vi "Search_From_Json.vi"(0 "Data JSON":string, 7 "ERD":string, 11 "error in":errorcluster) -> (4 "Name":string, 6 "Type":string, 8 "Size data":string, 10 "Hexa":string, 15 "error IO":errorcluster)   [LabVIEW 2021]
uses:
  <vilib>/JDP Science/JSONtext/Find Item.vi
  <vilib>/JDP Science/JSONtext/String Subset.vi
  <vilib>/JDP Science/JSONtext/Offset/Find Object Item Locations by Names.vi
  <vilib>/JDP Science/JSONtext/support/Quote and Escape JSON string.vi
  <vilib>/JDP Science/JSONtext/Next JSON Value.vi
  <vilib>/JDP Science/JSONtext/Parsing/Advance past whitespace.vi
  <vilib>/JDP Science/JSONtext/support/Commas Needed.vi
  <vilib>/JDP Science/JSONtext/Parsing/Advance past whitespace and comma.vi
  <vilib>/JDP Science/JSONtext/Parsing/Advance past next JSON Value (inlined COPY).vi
  <vilib>/JDP Science/JSONtext/Parsing/Advance past Item Name.vi
  <vilib>/JDP Science/JSONtext/support/quote and escape json string 2.vi
  <vilib>/JDP Science/JSONtext/Parsing/Advance past Line Ending.vi
  <vilib>/JDP Science/JSONtext/Parsing/Advance past String.vi
  <vilib>/JDP Science/JSONtext/Parsing/Advance past Number.vi
  <vilib>/JDP Science/JSONtext/Parsing/Parse Full Path or Item Name.vi
  <vilib>/JDP Science/JSONtext/Parsing/Advance past Array.vi
  <vilib>/JDP Science/JSONtext/Parsing/Advance past Object.vi
  <vilib>/JDP Science/JSONtext/support/Error Cluster From Code.vi
  <vilib>/JDP Science/JSONtext/Offset/Find Item Locations by Path.vi
  <vilib>/JDP Science/JSONtext/Parsing/Parsing Error.vi
  <vilib>/JDP Science/JSONtext/JSONtext.lvlib
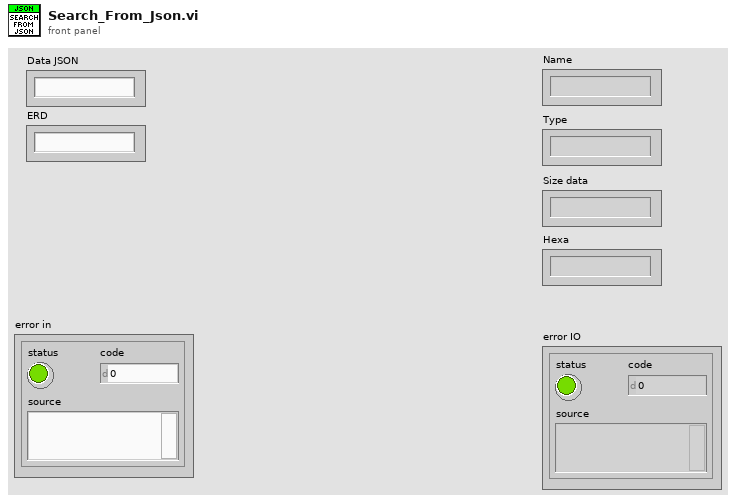
[diagram p1: front panel]
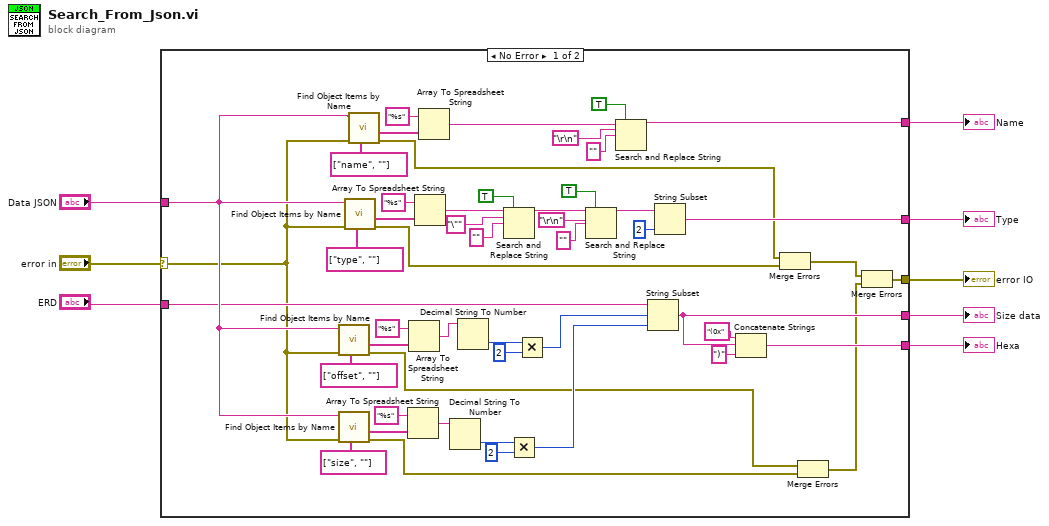
[diagram p0: block diagram]
diagram:
  n1 = case shown="No Error" "error in" {
    selector: "error in" -> [w16 w59]
    tunnel: "Data JSON" -> [w22 _]
    tunnel: "ERD" -> [w21 _]
    tunnel: [w20 _] -> w6
    tunnel: [w19 _] -> w5
    tunnel: [w18 _] -> w4
    tunnel: [w17 _] -> w3
    tunnel: [w9 w59] -> w1
    frame No Error {
      n2 = call <vilib>:"Find Object Items by Name.vi"("Item Names"=string[] ["offset", ""], "error in (no error)"=w16, "JSON"=w22) -> ("error out"=w14:errorcluster, "<JSON>"=w45:string[])  [unwired: 6 in, 1 out]
      n3 = call <vilib>:"Find Object Items by Name.vi"("Item Names"=string[] ["size", ""], "error in (no error)"=w16, "JSON"=w22) -> ("error out"=w15:errorcluster, "<JSON>"=w44:string[])  [unwired: 6 in, 1 out]
      n4 = call <vilib>:"Find Object Items by Name.vi"("Item Names"=string[] ["type", ""], "error in (no error)"=w16, "JSON"=w22) -> ("error out"=w12:errorcluster, "<JSON>"=w56:string[])  [unwired: 6 in, 1 out]
      n5 = call <vilib>:"Find Object Items by Name.vi"("Item Names"=string[] ["name", ""], "error in (no error)"=w16, "JSON"=w22) -> ("error out"=w13:errorcluster, "<JSON>"=w50:string[])  [unwired: 6 in, 1 out]
      n6 = Array To Spreadsheet String(array=w44, 3:"%s" ("format string")) -> (spreadsheet string=w43:string)  [unwired: 1 in]
      n7 = Array To Spreadsheet String(array=w45, 3:"%s" ("format string")) -> (spreadsheet string=w38:string)  [unwired: 1 in]
      n8 = Array To Spreadsheet String(array=w56, 3:"%s" ("format string")) -> (spreadsheet string=w35:string)  [unwired: 1 in]
      n9 = Array To Spreadsheet String(array=w50, 3:"%s" ("format string")) -> (spreadsheet string=w25:string)  [unwired: 1 in]
      n10 = Decimal String To Number(string=w43) -> (number=w42:i32)  [unwired: 2 in, 1 out]
      n11 = Decimal String To Number(string=w38) -> (number=w39:i32)  [unwired: 2 in, 1 out]
      n12 = Search and Replace String(replace all?=TRUE ("replace all? (F)"), input string=w35, search string="\"", replace string="" ("replace string (\"\")")) -> (result string=w34:string)  [unwired: 4 in, 3 out]
      n13 = Multiply(x=w42, y=2) -> (x*y=w36:i32)
      n14 = Multiply(x=w39, y=2) -> (x*y=w37:i32)
      n15 = Search and Replace String(replace all?=TRUE ("replace all? (F)"), input string=w34, search string="\r\n", replace string="" ("replace string (\"\")")) -> (result string=w30:string)  [unwired: 4 in, 3 out]
      n16 = Search and Replace String(replace all?=TRUE ("replace all? (F)"), input string=w25, search string="\r\n", replace string="" ("replace string (\"\")")) -> (result string=w17:string)  [unwired: 4 in, 3 out]
      n17 = String Subset(string=w21, offset (0)=w37, length (rest)=w36) -> (substring=w18:string)
      n18 = String Subset(string=w30, length (rest)=2 ("length (rest)")) -> (substring=w20:string)  [unwired: 1 in]
      n19 = Concatenate Strings("(0x" ("string"), w18, ")" ("string")) -> (w19:string)
      n20 = Merge Errors(w13, w12) -> (w11:errorcluster)
      n21 = Merge Errors(w14, w15) -> (w10:errorcluster)
      n22 = Merge Errors(w11, w10) -> (w9:errorcluster)
    }
    frame Error {
    }
  }
  "Type" <- w6
  "Hexa" <- w5
  "Size data" <- w4
  "Name" <- w3
  "error IO" <- w1
